vi "update scan specification.vi"(6 "auto-center scan":bool=TRUE, 7 "trigger":bool, 11 "scan specification":T1={"x amplitude"=1000, "x resolution (pixels)"=100, "x offset fly-forward (iterations)"=0, "x offset fly-back (iterations)"=0, "y resolution (nr. of lines)"=200, "y step size"=5, "iterations per pixel"=5, "number of frames"=-1, "y offset (pixels)"=0, "number of y-brake lines  (before y-fly-back)"=2, "number y-brake lines (after y-fly-back)"=2, "number of y-fly-back steps"=2, "lines per z step"=5, "number of z/intensity tuples"=200, "number of repetitions (volumes or planes)"=500, "z step size derived"=0, "choose the beginning of z scan"=FALSE, "number of frames (settings)"=0, "FPGA trajectory?"=FALSE}) -> (3 "scan specification out":T1={"x amplitude"=1000, "x resolution (pixels)"=100, "x offset fly-forward (iterations)"=0, "x offset fly-back (iterations)"=0, "y resolution (nr. of lines)"=200, "y step size"=5, "iterations per pixel"=5, "number of frames"=-1, "y offset (pixels)"=0, "number of y-brake lines  (before y-fly-back)"=2, "number y-brake lines (after y-fly-back)"=2, "number of y-fly-back steps"=2, "lines per z step"=5, "number of z/intensity tuples"=200, "number of repetitions (volumes or planes)"=500, "z step size derived"=0, "choose the beginning of z scan"=FALSE, "number of frames (settings)"=0, "FPGA trajectory?"=FALSE})   [LabVIEW 2010]
uses:
  scan_specification_cluster.ctl
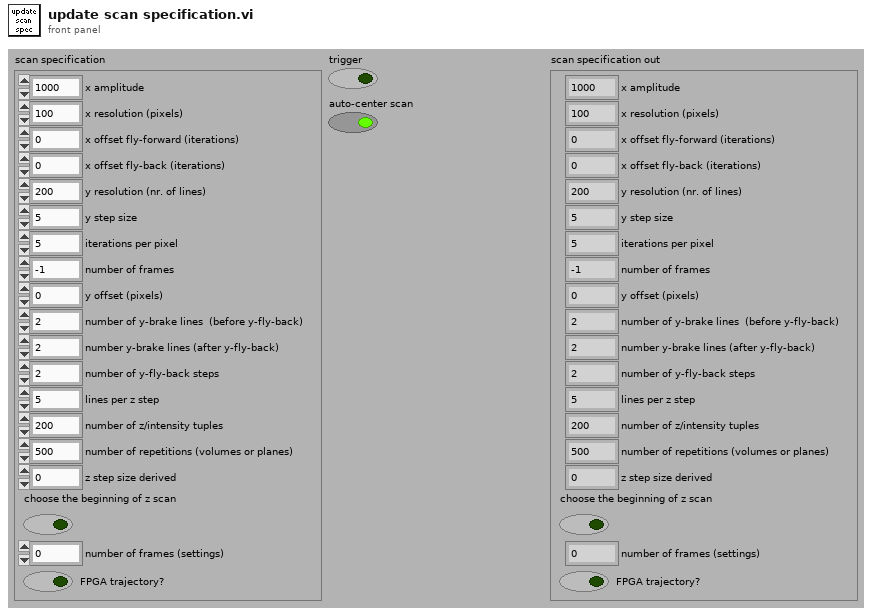
[diagram p1: front panel]
types:
  T1 = typedef "scan_specification_cluster.ctl" = cluster{"x amplitude":u16, "x resolution (pixels)":u16, "x offset fly-forward (iterations)":u16, "x offset fly-back (iterations)":u16, "y resolution (nr. of lines)":u16, "y step size":u16, "iterations per pixel":u16, "number of frames":i32, "y offset (pixels)":u16, "number of y-brake lines  (before y-fly-back)":u16, "number y-brake lines (after y-fly-back)":u16, "number of y-fly-back steps":u16, "lines per z step":u16, "number of z/intensity tuples":u16, "number of repetitions (volumes or planes)":i32, "z step size derived":u16, "choose the beginning of z scan":bool, "number of frames (settings)":i32, "FPGA trajectory?":bool}
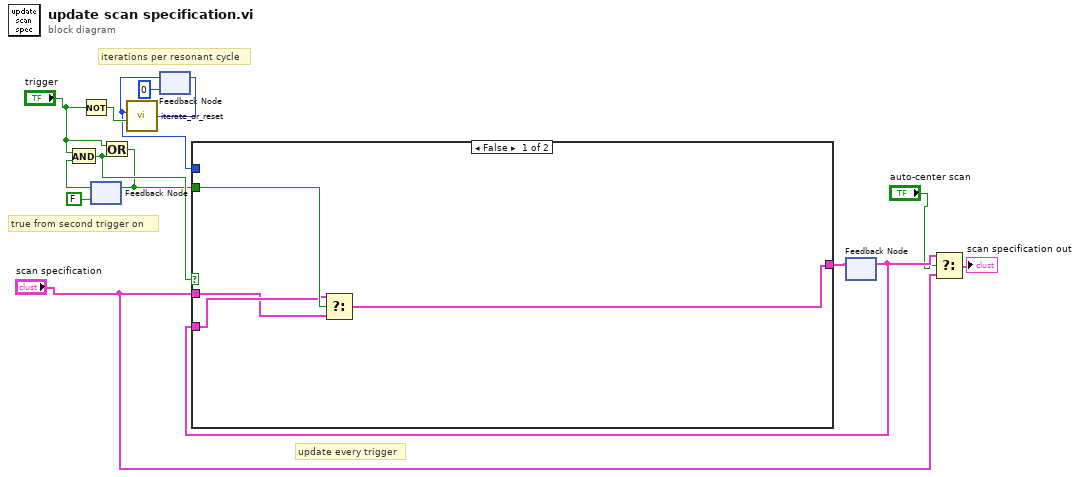
[diagram p0: block diagram]
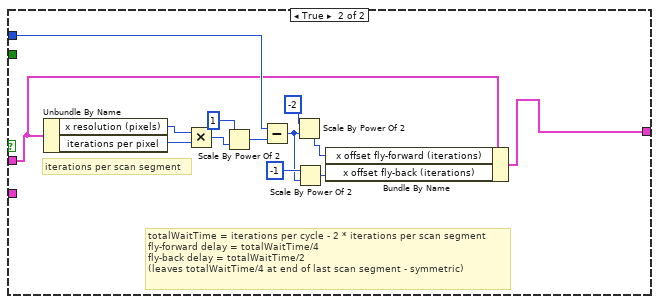
[diagram p2: hidden frame]
diagram:
  # "update every trigger"
  # "true from second trigger on"
  # "iterations per resonant cycle"
  n1 = Not(x="trigger") -> (.not. x?=w14:bool)
  n2 = feedback #1(FALSE) -> (w11:bool)
  n3 = And(x="trigger", y=w11) -> (x .and. y?=w9:bool)
  n4 = Or(x="trigger", y=w9) -> (x .or. y?=w5:bool)
  n5 = feedback-in #1(w5) -> ()
  n6 = feedback #2(u16 0 ("number out")) -> (w7:u16)
  n7 = call "iterate_or_reset.vi"("iterate?"=w14, "number in"=w7) -> ("number out"=w8:u16)  [unwired: 4 in]
  n8 = feedback-in #2(w8) -> ()
  n9 = feedback #3() -> (w3:T1)  [unwired: 1 in]
  n10 = case shown="False" w9 {
    tunnel: w7 -> [_ w28]
    tunnel: "scan specification" -> [w16 w24]
    tunnel: [w15 w19] -> w6
    tunnel: w3 -> [w17 _]
    tunnel: w5 -> [w18 _]
    frame False {
      n11 = Select(t=w17, s=w18, f=w16) -> (s? t:f=w15:T1)
    }
    frame True {
      # "totalWaitTime = iterations per cycle - 2 * iterations per scan segment\nfly-forward delay = totalWaitTime/4\nfly-back delay = totalWaitTime/2 \n(leaves totalWaitTime/4 at end of last scan segment - symmetric)"
      # "iterations per scan segment"
      n12 = Unbundle By Name(w24) -> ("x resolution (pixels)"=w31:u16, "iterations per pixel"=w30:u16)
      n13 = Multiply(x=w31, y=w30) -> (x*y=w27:u16)
      n14 = Scale By Power Of 2(n=u16 1 ("x"), x=w27) -> (x*2^n=w29:u16)
      n15 = Subtract(x=w28, y=w29) -> (x-y=w22:u16)
      n16 = Scale By Power Of 2(n=-2, x=w22) -> (x*2^n=w21:u16)
      n17 = Scale By Power Of 2(n=i16 -1, x=w22) -> (x*2^n=w20:u16)
      n18 = Bundle By Name(cluster=w24, "x offset fly-forward (iterations)"=w21, "x offset fly-back (iterations)"=w20) -> (w19:T1)
    }
  }
  n19 = feedback-in #3(w6) -> ()
  n20 = Select(t=w3, s="auto-center scan", f="scan specification") -> (s? t:f=→"scan specification out":T1)
